vi "Agilent E364X Series Output Single Channel DC Volts.vi"(0 "VISA resource name":refnum<visa-resource-name>, 1 "Output Enabled (False)":bool, 5 "Voltage Level (0.0 Volts)":dbl format="%.2p", 7 "Current Limit (0 Amps)":dbl format="%.2p", 9 "OVP Limit (22.0 Volts)":dbl=22.0 format="%.2p", 11 "error in (no error)":errorcluster, 12 "OVP Enabled (True)":bool=TRUE) -> (6 "Over Voltage Protection":bool)   [LabVIEW 2013]
doc: "This VI configures the specifies power supply's channel to generate a DC voltage by taking the following steps:\n\n1) Configure current limit.\n\n2) Configure the over voltage protection.\n\n3) Configure the voltage level.\n\n4) Enable or disable the power output.\n\n5) Query the over voltage output state.\n\nNotes:\n\n(1) This VI takes a couple seconds to finish so that it may correctly get the current OVP value."
uses:
  <instrlib>/Agilent E364X Series/Agilent E364X Series.lvlib
panel:
  # "© 2005 National Instruments.  ALL RIGHTS RESERVED."
  # "For instructions,\nselect Show Context Help\nfrom the Help menu."
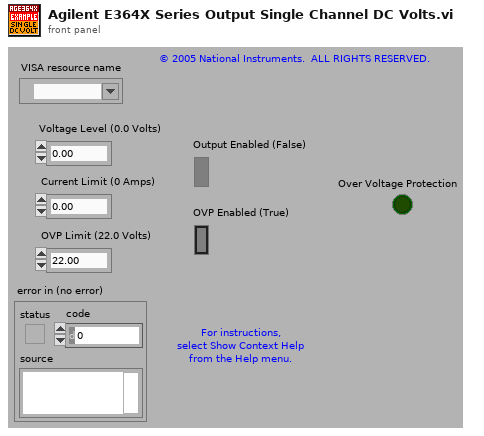
[diagram p1: front panel]
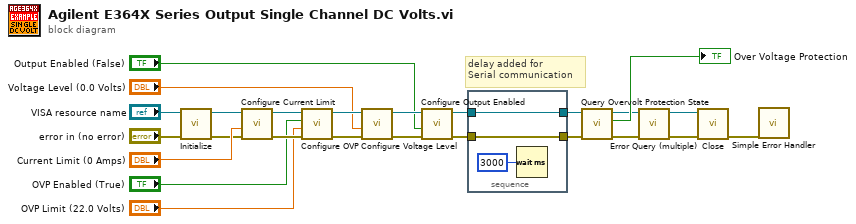
[diagram p0: block diagram]
diagram:
  # "delay added for \nSerial communication"
  n1 = call "Initialize.vi"("error in (no error)"="error in (no error)", "VISA resource name"="VISA resource name") -> ("error out"=w1:errorcluster, "VISA resource name out"=w2:refnum<visa-resource-name>)  [unwired: 8 in]
  n2 = call "Configure Current Limit.vi"("error in (no error)"=w1, "Current Limit (0.0 Amps)"="Current Limit (0 Amps)", "VISA resource name"=w2) -> ("error out"=w25:errorcluster, "VISA resource name out"=w24:refnum<visa-resource-name>)  [unwired: 7 in]
  n3 = call "Configure OVP.vi"("error in (no error)"=w25, "Limit (22.0 Volts)"="OVP Limit (22.0 Volts)", "OVP Enabled (T: On)"="OVP Enabled (True)", "VISA resource name"=w24) -> ("error out"=w21:errorcluster, "VISA resource name out"=w22:refnum<visa-resource-name>)  [unwired: 6 in]
  n4 = call "Configure Voltage Level.vi"("error in (no error)"=w21, "Level (0.0 Volts)"="Voltage Level (0.0 Volts)", "VISA resource name"=w22) -> ("error out"=w18:errorcluster, "VISA resource name out"=w19:refnum<visa-resource-name>)  [unwired: 7 in]
  n5 = call "Configure Output Enabled.vi"("error in (no error)"=w18, "Output Enabled (F: Off)"="Output Enabled (False)", "VISA resource name"=w19) -> ("error out"=w13:errorcluster, "VISA resource name out"=w14:refnum<visa-resource-name>)  [unwired: 7 in]
  n6 = stacked-sequence {
    tunnel: w14 -> [w27]
    tunnel: w13 -> [w26]
    tunnel: [w27] -> w12
    tunnel: [w26] -> w11
    frame #0 {
      n7 = Wait (ms)(milliseconds to wait=u32 3000) -> ()  [unwired: 1 out]
    }
  }
  n8 = call "Query Overvolt Protection State.vi"("error in (no error)"=w11, "VISA resource name"=w12) -> ("error out"=w8:errorcluster, "Over Voltage Protection"=→"Over Voltage Protection":bool, "VISA resource name out"=w9:refnum<visa-resource-name>)  [unwired: 7 in]
  n9 = call "Error Query (multiple).vi"("error in (no error)"=w8, "VISA resource name"=w9) -> ("error out"=w6:errorcluster, "VISA resource name out"=w7:refnum<visa-resource-name>)  [unwired: 6 in, 2 out]
  n10 = call "Close.vi"("error in (no error)"=w6, "VISA resource name"=w7) -> ("error out"=w5:errorcluster)  [unwired: 9 in]
  n11 = call <vilib>:"Simple Error Handler.vi"("error in (no error)"=w5) -> ()  [unwired: 4 in, 5 out]
